vi "MeasLink Plugin Path.vi"(11 "error in (no error)":errorcluster) -> (0 "Measurement UI Lib":path, 1 "Run Service":path, 2 "Measurement UI":path, 3 "Instrumentstudio Folder":path, 4 "New Code Module":path, 5 "Set Default Value":path, 6 "Wrapper Path":path, 8 "Result Control":path, 10 "Input Controls":path, 12 "Library":path, 13 "Type Specialization":path, 14 "Logic VI Path":path, 15 "error out":errorcluster)   [LabVIEW 2021, in "Path Functions.lvlib"]
uses:
  Path Functions.lvlib
  Migrator Reusables/Migrator Reusables.lvlib
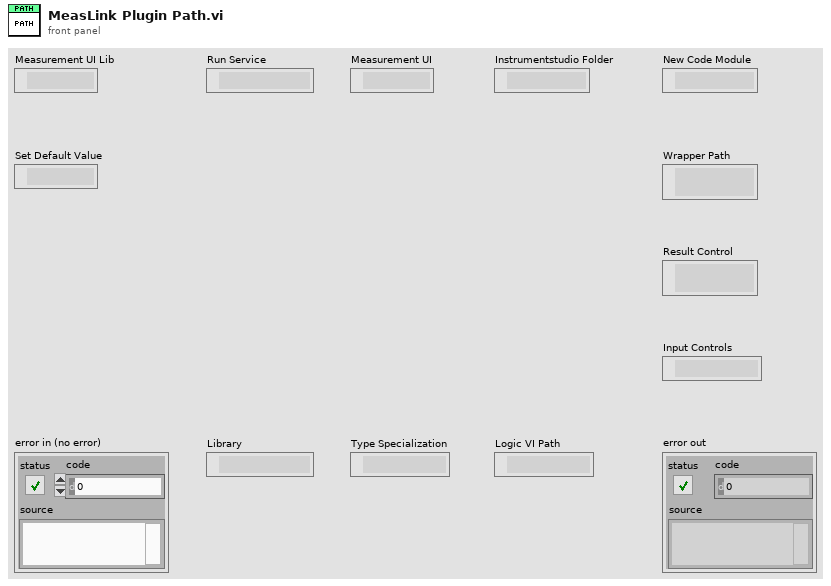
[diagram p1: front panel]
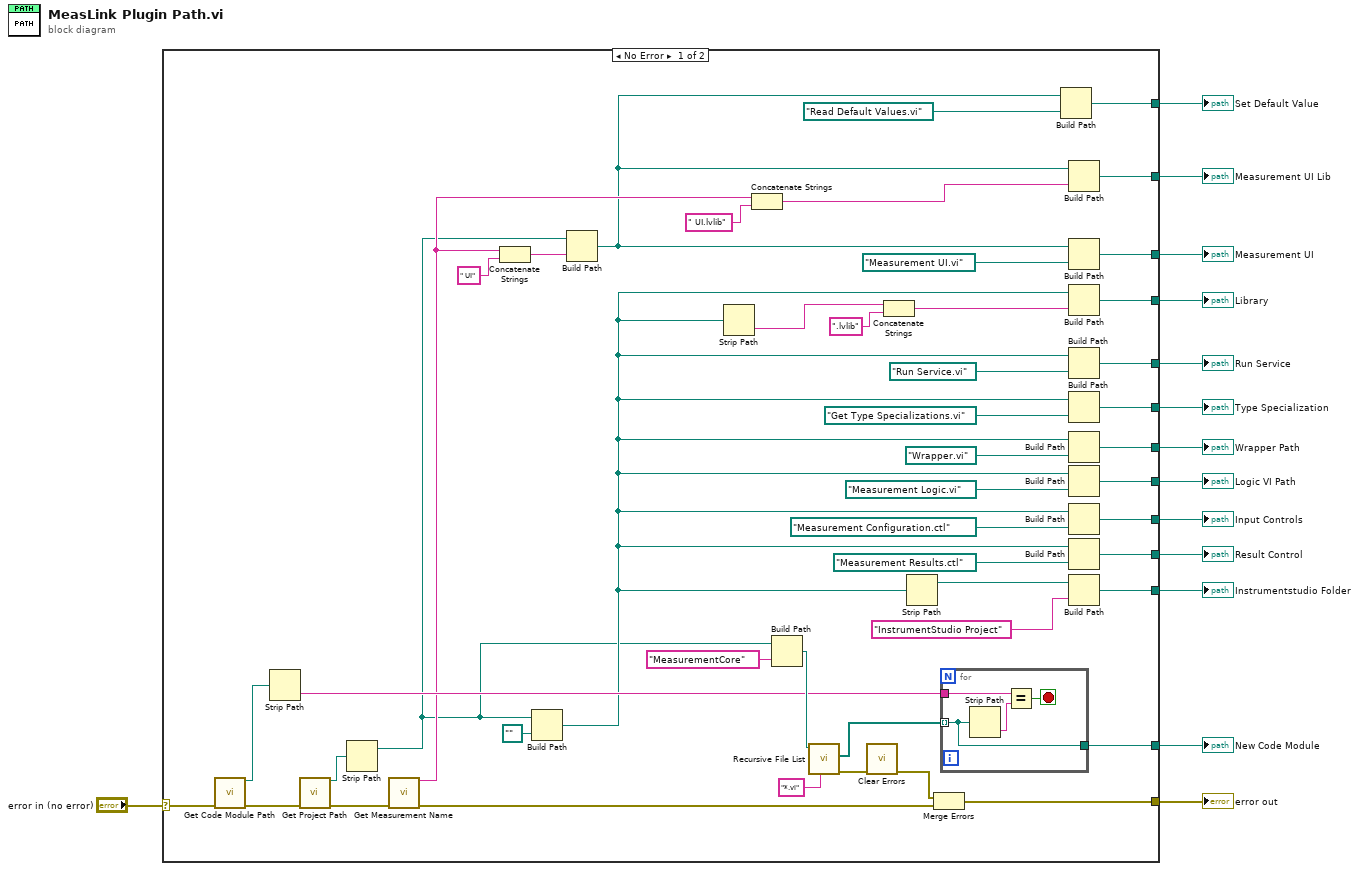
[diagram p0: block diagram]
diagram:
  n1 = case shown="No Error" "error in (no error)" {
    selector: "error in (no error)" -> [w43 w67]
    tunnel: [w62 _] -> w14
    tunnel: [w61 _] -> w13
    tunnel: [w60 _] -> w12
    tunnel: [w59 _] -> w11
    tunnel: [w53 _] -> w10
    tunnel: [w52 _] -> w9
    tunnel: [w50 _] -> w8
    tunnel: [w46 _] -> w7
    tunnel: [w39 _] -> w5
    tunnel: [w28 w67] -> w4
    tunnel: [w27 _] -> w3
    tunnel: [w20 _] -> w2
    tunnel: [w19 _] -> w1
    frame No Error {
      n2 = call "Get Code Module Path.vi"("error in (no error)"=w43) -> ("CodeModule Out"=w41:path, "error out"=w42:errorcluster)  [unwired: 13 in]
      n3 = Strip Path(path=w41) -> (name=w30:string)  [unwired: 1 out]
      n4 = call "Get Project Path.vi"("error in (no error)"=w42) -> ("Project Path Out"=w45:path, "error out"=w44:errorcluster)  [unwired: 13 in]
      n5 = Strip Path(path=w45) -> (stripped path=w16:path)  [unwired: 1 out]
      n6 = call "Get Measurement Name.vi"("error in (no error)"=w44) -> ("Name Out"=w21:string, "error out"=w29:errorcluster)  [unwired: 13 in]
      n7 = Concatenate Strings(w21, " UI" ("string")) -> (w24:string)
      n8 = Build Path(base path=w16, name or relative path=path "") -> (appended path=w26:path)
      n9 = Build Path(base path=w16, name or relative path=w24) -> (appended path=w18:path)
      n10 = Strip Path(path=w26) -> (name=w40:string)  [unwired: 1 out]
      n11 = Concatenate Strings(w21, " UI.lvlib" ("string")) -> (w22:string)
      n12 = Build Path(base path=w16, name or relative path="MeasurementCore" ("string")) -> (appended path=w33:path)
      n13 = call <vilib>:"Recursive File List.vi"("pattern"="*.vi", "Folder Path"=w33) -> ("error out"=w32:errorcluster, "All Files in Dir"=w34:path[])  [unwired: 5 in, 3 out]
      n14 = call <vilib>:"Clear Errors.vi"("error in (no error)"=w32) -> ("error out"=w31:errorcluster)  [unwired: 5 in, 1 out]
      n15 = Concatenate Strings(w40, ".lvlib" ("string")) -> (w38:string)
      n16 = Strip Path(path=w26) -> (stripped path=w49:path)  [unwired: 1 out]
      n17 = Merge Errors(w31, w29) -> (w28:errorcluster)
      n18 = for {
        tunnel: w34 -> [w64] mode=indexing
        tunnel: w30 -> [w66]
        tunnel: [w64] -> w27
        stop <- w63 stop-if-true
        n19 = Strip Path(path=w64) -> (name=w65:string)  [unwired: 1 out]
        n20 = Equal?(x=w66, y=w65) -> (x = y?=w63:bool)
      }
      n21 = Build Path(base path=w18, name or relative path=path "Read Default Values.vi") -> (appended path=w19:path)
      n22 = Build Path(base path=w18, name or relative path=w22) -> (appended path=w20:path)
      n23 = Build Path(base path=w18, name or relative path=path "Measurement UI.vi") -> (appended path=w53:path)
      n24 = Build Path(base path=w26, name or relative path=w38) -> (appended path=w39:path)
      n25 = Build Path(base path=w26, name or relative path=path "Run Service.vi") -> (appended path=w46:path)
      n26 = Build Path(base path=w26, name or relative path=path "Get Type Specializations.vi") -> (appended path=w52:path)
      n27 = Build Path(base path=w26, name or relative path=path "Wrapper.vi") -> (appended path=w62:path)
      n28 = Build Path(base path=w26, name or relative path=path "Measurement Logic.vi") -> (appended path=w61:path)
      n29 = Build Path(base path=w26, name or relative path=path "Measurement Configuration.ctl") -> (appended path=w60:path)
      n30 = Build Path(base path=w26, name or relative path=path "Measurement Results.ctl") -> (appended path=w59:path)
      n31 = Build Path(base path=w49, name or relative path="InstrumentStudio Project" ("string")) -> (appended path=w50:path)
    }
    frame Error {
    }
  }
  "error out" <- w4
  "New Code Module" <- w3
  "Wrapper Path" <- w14
  "Logic VI Path" <- w13
  "Input Controls" <- w12
  "Result Control" <- w11
  "Instrumentstudio Folder" <- w8
  "Measurement UI" <- w10
  "Type Specialization" <- w9
  "Run Service" <- w7
  "Library" <- w5
  "Measurement UI Lib" <- w2
  "Set Default Value" <- w1
